vi "Scanimage Query.vi"(8 "error in":errorcluster, 10 "query":string, 11 "port":string) -> (0 "error out":errorcluster, 2 "Response":string, 3 "port out":string)   [LabVIEW 2012, in "Sciscan Scope Daemon.lvlib"]
uses:
  Sciscan Scope Daemon.lvlib
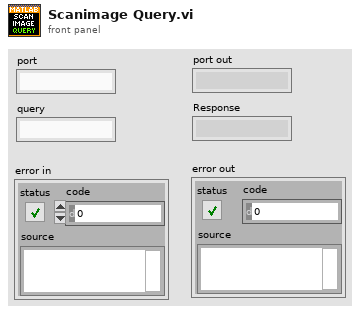
[diagram p1: front panel]
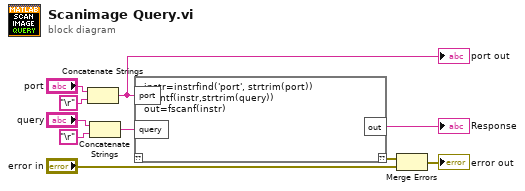
[diagram p0: block diagram]
diagram:
  n1 = Concatenate Strings("port", "\r") -> (w7:string)
  "port out" <- w7
  n2 = Concatenate Strings("query", "\r") -> (w5:string)
  n3 = script code="instr=instrfind('port', strtrim(port))\nfprintf(instr,strtrim(query))\nout=fscanf(instr)"("query"=w5, "port"=w7) -> ("??"=w2:errorcluster, "out"=→"Response":string)  [unwired: 1 in]
  n4 = Merge Errors(w2, "error in") -> (→"error out":errorcluster)
